vi "Send Set Relay Control Msg.vi"(8 "error in":errorcluster, 10 "Relay_Control":T1, 11 "SCADA Sub Abstract in":refnum<class "Device Communication and Control Abstract.lvclass">) -> (0 "error out":errorcluster, 3 "dup SCADA Sub Abstract":refnum<class "Device Communication and Control Abstract.lvclass">)   [LabVIEW 2018, in "Device Communication and Control Abstract Actor.lvlib" / "Device Communication and Control Abstract.lvclass"]
uses:
  Device Communication and Control Abstract.lvclass
  C:/Program Files (x86)/National Instruments/LabVIEW 2018/vi.lib/ActorFramework/Actor/Actor.lvclass
  <vilib>/ORNL/CSEISMIC DDS/CSEISMIC DDS Base/Data Types/Relay_Control.ctl
  <vilib>/ORNL/CSEISMIC DDS/CSEISMIC DDS Base/Data Types/Controls/DeviceID.ctl
  <vilib>/ActorFramework/Actor/Actor.lvclass/Actor.ctl
  Device Communication and Control Abstract.lvclass/Device Communication and Control Abstract.ctl
  Device Communication and Control Abstract Messages/Set Relay Control Msg/Set Relay Control Msg.lvclass/Set Relay Control Msg.ctl
  <vilib>/ActorFramework/Message Enqueuer/Message Enqueuer.lvclass/Message Enqueuer.ctl
  <vilib>/ActorFramework/Message Enqueuer/Enqueue.vi
  Device Communication and Control Abstract Messages/Set Relay Control Msg/Set Relay Control Msg.lvclass
  C:/Program Files (x86)/National Instruments/LabVIEW 2018/vi.lib/ActorFramework/Message/Message.lvclass
  <vilib>/ActorFramework/Message Priority Queue/Priority Enqueue.vi
  <vilib>/ActorFramework/Actor/Actor.lvclass
  <vilib>/ORNL/CSEISMIC DDS/CSEISMIC DDS Base/CSEISMIC DDS.lvclass
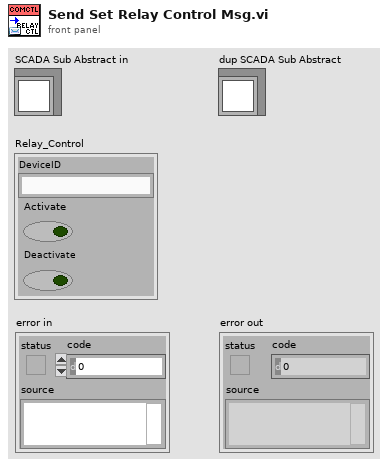
[diagram p1: front panel]
types:
  T1 = typedef "CSEISMIC DDS.lvlib/CSEISMIC DDS.lvclass/Relay_Control.ctl" = cluster{"DeviceID":T2, "Activate":bool, "Deactivate":bool}
  T2 = typedef "CSEISMIC DDS.lvlib/CSEISMIC DDS.lvclass/DeviceID.ctl" = string
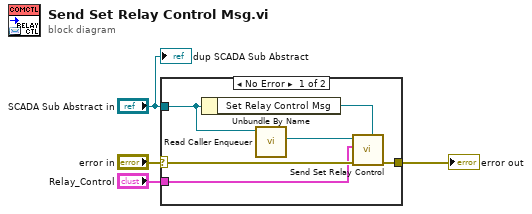
[diagram p0: block diagram]
diagram:
  n1 = case shown="No Error" "error in" {
    selector: "error in" -> [w10 w11]
    tunnel: "SCADA Sub Abstract in" -> [w6 _]
    tunnel: "Relay_Control" -> [w5 _]
    tunnel: [w9 w11] -> w1
    frame No Error {
      n2 = Unbundle By Name(w6) -> ("Set Relay Control Msg"=w8:refnum<class "Set Relay Control Msg.lvclass">)
      n3 = call <vilib>:"Read Caller Enqueuer.vi"("Actor"=w6) -> ("Caller Enqueuer"=w7:refnum<class "Message Enqueuer.lvclass">)  [unwired: 10 in]
      n4 = call "Send Set Relay Control.vi"("Message Type"=w8, "error in (no error)"=w10, "Relay_Control"=w5, "Message Enqueuer"=w7) -> ("error out"=w9:errorcluster)  [unwired: 6 in, 1 out]
    }
    frame Error {
    }
  }
  "error out" <- w1
  "dup SCADA Sub Abstract" <- "SCADA Sub Abstract in"
